vi "HAILO_packet_calibration.vi"(8 "Zero?":bool, 9 "Sensor Readings (Signed)":i16[](array[numeric])) -> (1 "F Shear":dbl[](array[numeric]), 2 "F Normal":dbl[](array[numeric]), 3 "Sensor Readings":dbl[][](array[numeric])=[[-533.0, -111.0, 239.0], [-402.0, 166.0, 184.0], [-184.0, 154.0, 29.0], [-106.0, 74.0, 11.0], [-532.0, -109.0, 246.0], [-398.0, 164.0, 175.0], [-205.0, 152.0, 32.0], [-119.0, 65.0, 9.0], [-529.0, -110.0, 242.0], [-408.0, 166.0, 184.0], [-198.0, 158.0, 27.0], [-108.0, 61.0, 6.0], [-539.0, -106.0, 240.0], [-407.0, 158.0, 183.0], [-191.0, 156.0, 28.0], [-113.0, 73.0, 15.0], [816.0, -260.0, 842.0], [539.0, 512.0, 512.0], [156.0, 425.0, 83.0], [13.0, 142.0, -72.0], [816.0, -262.0, 840.0], [528.0, 520.0, 512.0], [162.0, 425.0, 83.0], [13.0, 137.0, -84.0], [809.0, -260.0, 840.0], [538.0, 520.0, 504.0], [162.0, 432.0, 72.0], [13.0, 136.0, -84.0], [809.0, -260.0, 846.0], [538.0, 508.0, 512.0], [158.0, 435.0, 72.0], [19.0, 136.0, -79.0], [346.0, -168.0, 14.0], [287.0, -68.0, 19.0], [161.0, -34.0, 4.0], [70.0, -44.0, -7.0], [345.0, -191.0, 19.0], [279.0, -40.0, 8.0], [167.0, -16.0, 12.0], [72.0, -23.0, 2.0], [341.0, -190.0, 17.0], [285.0, -46.0, 9.0], [149.0, -15.0, 6.0], [54.0, -40.0, -2.0], [375.0, -201.0, 19.0], [282.0, -51.0, 10.0], [135.0, -37.0, 6.0], [81.0, -57.0, -12.0], [-80.0, -193.0, -48.0], [-73.0, -136.0, -12.0], [-5.0, -122.0, -31.0], [-19.0, -118.0, -17.0], [-118.0, -187.0, -48.0], [-73.0, -115.0, -22.0], [1.0, -113.0, -27.0], [-20.0, -111.0, -8.0], [-99.0, -184.0, -40.0], [-62.0, -145.0, -17.0], [0.0, -113.0, -37.0], [-7.0, -117.0, -15.0], [-126.0, -184.0, -50.0], [-72.0, -115.0, -14.0], [-4.0, -114.0, -25.0], [-29.0, -116.0, -14.0]])   [LabVIEW 2016]
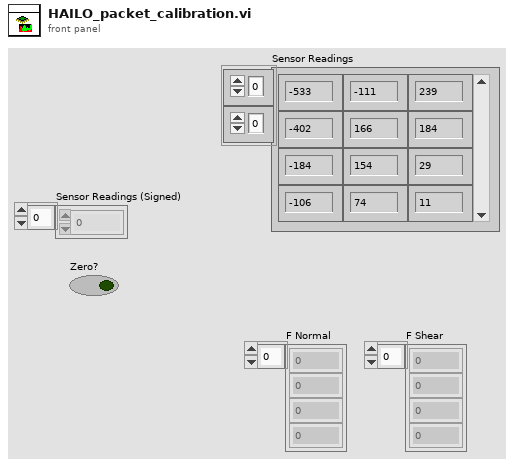
[diagram p1: front panel]
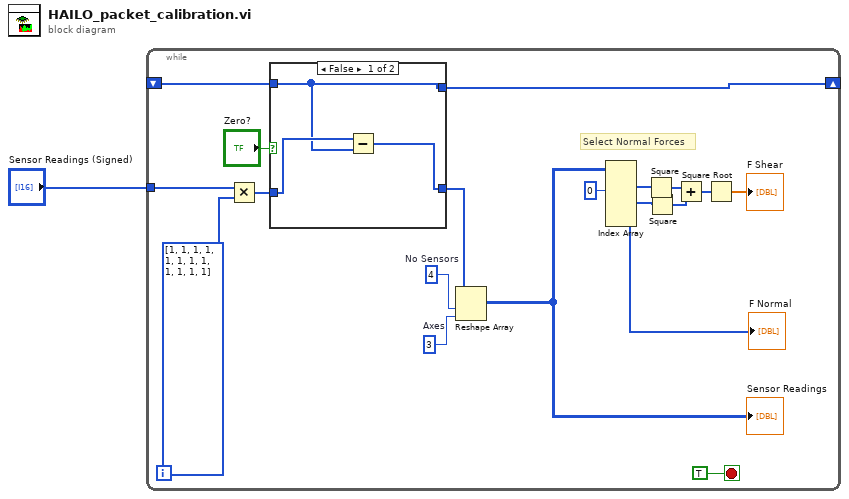
[diagram p0: block diagram]
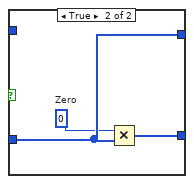
[diagram p2: hidden frame]
diagram:
  n1 = while {
    tunnel: "Sensor Readings (Signed)" -> [w17]
    shift-right: [w12] -> _
    shift-left: _ -> [w13]
    stop <- TRUE stop-if-true
    w19 = 4  # No Sensors
    w20 = 3  # Axes
    # "Select Normal Forces"
    n2 = Multiply(x=w17, y=i16[] [1, 1, 1, 1, 1, 1, 1, 1, 1, 1, 1, 1]) -> (x*y=w14:i16[])
    n3 = case shown="False" "Zero?" {
      tunnel: w14 -> [w23 w26]
      tunnel: w13 -> [w21 _]
      tunnel: [w21 w26] -> w12
      tunnel: [w22 w25] -> w11
      frame False {
        n4 = Subtract(x=w23, y=w21) -> (x-y=w22:i16[])
      }
      frame True {
        w24 = 0  # Zero
        n5 = Multiply(x=w24, y=w26) -> (x*y=w25:i32[])
      }
    }
    n6 = Reshape Array(w11, w19, w20) -> (w9:i32[][])
    "Sensor Readings" <- w9
    n7 = Index Array(array=w9, index (col) #1=0 ("disabled index (col)")) -> (element #1=w7:i32[], element #2=w6:i32[], element #3=→"F Normal":i32[])  [unwired: 5 in]
    n8 = Square(x=w7) -> (x^2=w5:i32[])
    n9 = Square(x=w6) -> (x^2=w4:i32[])
    n10 = Add(x=w5, y=w4) -> (x+y=w3:i32[])
    n11 = Square Root(x=w3) -> (sqrt(x)=→"F Shear":dbl[])
  }
